vi "QUIZ 1.vi"() -> ()   [LabVIEW 2019]
panel:
  out "Control de pertenencia de la coordenada":bool
  in  "Coordenada Y del punto":dbl[](array[numeric])
  out "Gráfica":T1(graph)
  in  "Coordenada X del punto":dbl[](array[numeric])
  in  "Y polinomio":dbl[](array[numeric])
  in  "X polinomio":dbl[](array[numeric])
  out "By":dbl[](array[numeric])
  out "Bx":dbl[](array[numeric])
  out "Ay":dbl[](array[numeric])
  out "Ax":dbl[](array[numeric])
  out "sum":dbl
  out "Angulos":dbl[](array[numeric])
  # "JOSE IVAN MENDEZ CORREA"
  # "MATEO CARO ROJO"
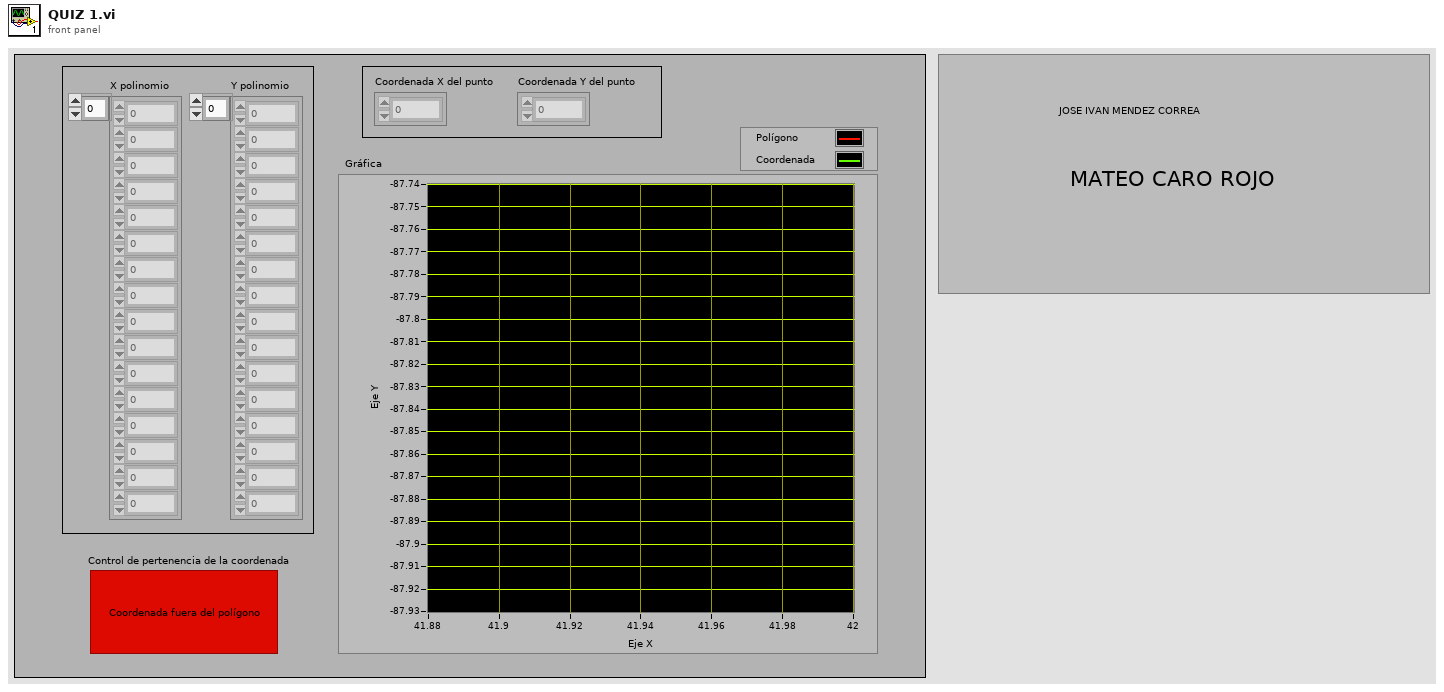
[diagram p1: front panel]
types:
  T1 = cluster{"coordenada X del punto":dbl[], "coordenada y del punto":dbl[]}[]
  T2 = cluster{"X polinomio":dbl[], "Y polinomio":dbl[]}
  T3 = cluster{"Coordenada X del punto":dbl[], "Coordenada Y del punto ":dbl[]}
  T4 = cluster{"Coordenada X del punto":dbl[], "Coordenada Y del punto ":dbl[]}[]
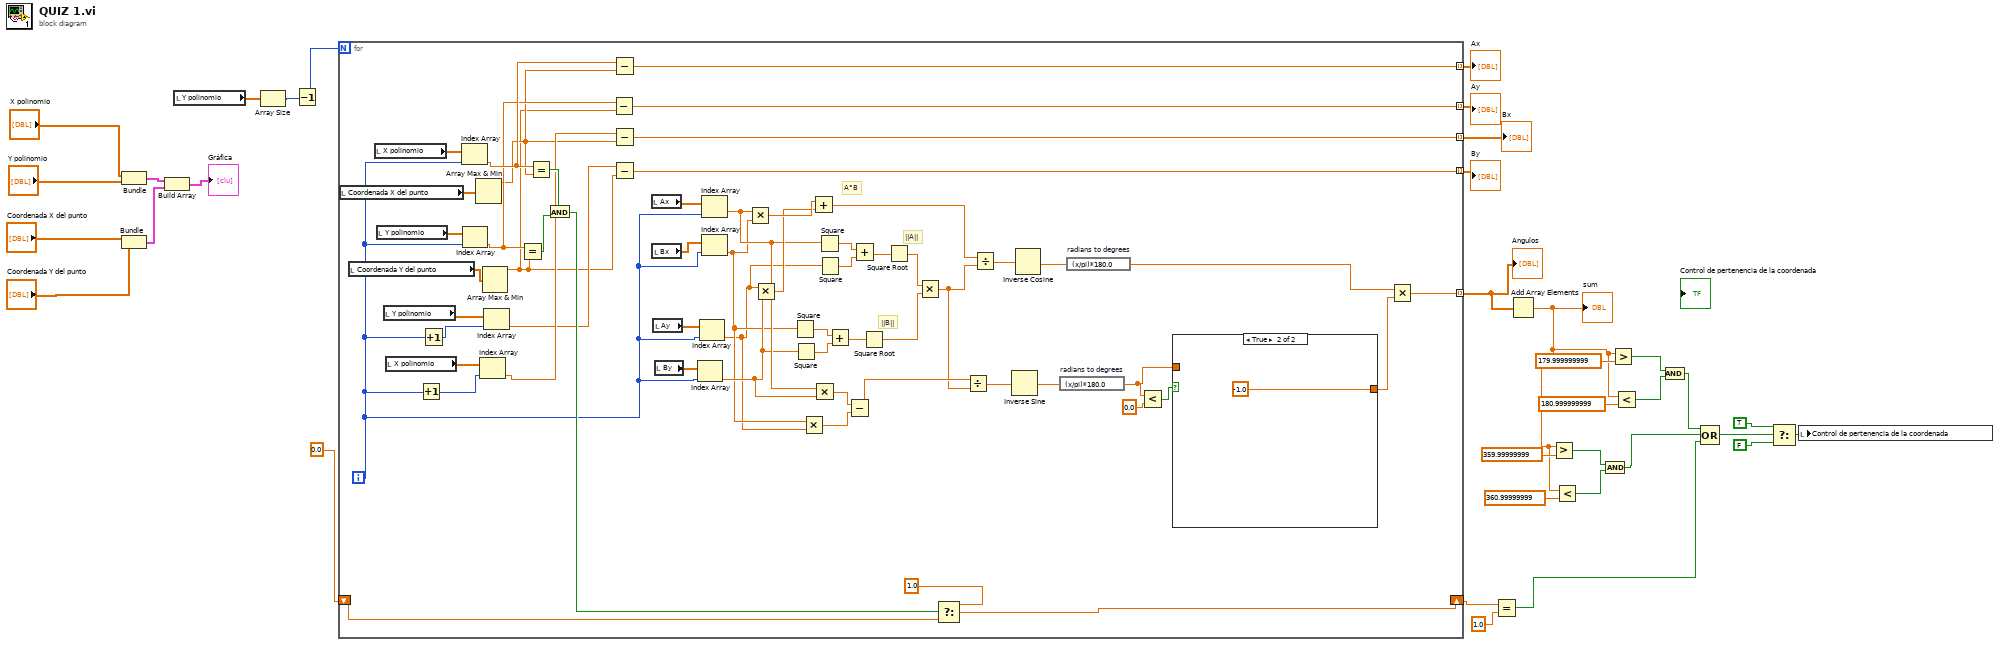
[diagram p0: block diagram]
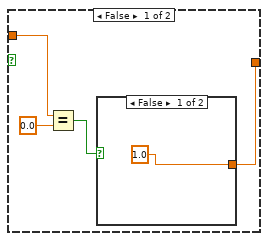
[diagram p2: hidden frame]
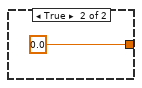
[diagram p3: hidden frame]
diagram:
  n1 = Bundle("X polinomio"="X polinomio", "Y polinomio"="Y polinomio") -> (w32:T2)  [unwired: 1 in]
  n2 = Bundle("Coordenada X del punto"="Coordenada X del punto", "Coordenada Y del punto"="Coordenada Y del punto") -> (w31:T3)  [unwired: 1 in]
  n3 = Build Array(w32, w31) -> (→"Gráfica":T4)
  n4 = local read "Y polinomio"() -> (w27:dbl[])
  n5 = Array Size(array=w27) -> (size(s)=w22:i32)
  n6 = Decrement(x=w22) -> (x-1=w23:i32)
  n7 = for {
    N: w23 -> [_]
    shift-right: [w83] -> w25
    shift-left: 0.0 -> [w86]
    tunnel: [w77] -> w21 mode=indexing
    tunnel: [w75] -> w20 mode=indexing
    tunnel: [w70] -> w19 mode=indexing
    tunnel: [w69] -> w18 mode=indexing
    tunnel: [w35] -> w17 mode=indexing
    i -> [w64]
    # "||B||"
    # "||A||"
    # "A°B"
    n8 = local read "Coordenada X del punto"() -> (w88:dbl[])
    n9 = local read "Coordenada Y del punto"() -> (w87:dbl[])
    n10 = local read "X polinomio"() -> (w92:dbl[])
    n11 = local read "Y polinomio"() -> (w91:dbl[])
    n12 = local read "Y polinomio"() -> (w82:dbl[])
    n13 = local read "X polinomio"() -> (w80:dbl[])
    n14 = Increment(x=w64) -> (x+1=w79:i32)
    n15 = Increment(x=w64) -> (x+1=w81:i32)
    n16 = Index Array(array=w92, index=w64) -> (element=w78:dbl)
    n17 = Index Array(array=w91, index=w64) -> (element=w76:dbl)
    n18 = Array Max & Min(array=w88) -> (max value=w73:dbl)  [unwired: 3 out]
    n19 = Index Array(array=w80, index=w79) -> (element=w74:dbl)
    n20 = Array Max & Min(array=w87) -> (max value=w71:dbl)  [unwired: 3 out]
    n21 = Index Array(array=w82, index=w81) -> (element=w72:dbl)
    n22 = Equal?(x=w76, y=w71) -> (x = y?=w89:bool)
    n23 = Equal?(x=w78, y=w73) -> (x = y?=w90:bool)
    n24 = And(x=w90, y=w89) -> (x .and. y?=w84:bool)
    n25 = Subtract(x=w76, y=w71) -> (x-y=w75:dbl)
    n26 = Subtract(x=w78, y=w73) -> (x-y=w77:dbl)
    n27 = Subtract(x=w74, y=w73) -> (x-y=w70:dbl)
    n28 = Subtract(x=w72, y=w71) -> (x-y=w69:dbl)
    n29 = local read "Ax"() -> (w68:dbl[])
    n30 = local read "Bx"() -> (w67:dbl[])
    n31 = local read "Ay"() -> (w66:dbl[])
    n32 = local read "By"() -> (w65:dbl[])
    n33 = Index Array(array=w65, index=w64) -> (element=w49:dbl)
    n34 = Index Array(array=w66, index=w64) -> (element=w47:dbl)
    n35 = Index Array(array=w68, index=w64) -> (element=w50:dbl)
    n36 = Index Array(array=w67, index=w64) -> (element=w48:dbl)
    n37 = Multiply(x=w50, y=w48) -> (x*y=w63:dbl)
    n38 = Multiply(x=w47, y=w49) -> (x*y=w62:dbl)
    n39 = Square(x=w48) -> (x^2=w58:dbl)
    n40 = Square(x=w49) -> (x^2=w57:dbl)
    n41 = Multiply(x=w48, y=w47) -> (x*y=w45:dbl)
    n42 = Add(x=w63, y=w62) -> (x+y=w53:dbl)
    n43 = Multiply(x=w50, y=w49) -> (x*y=w46:dbl)
    n44 = Square(x=w50) -> (x^2=w61:dbl)
    n45 = Square(x=w47) -> (x^2=w60:dbl)
    n46 = Add(x=w58, y=w57) -> (x+y=w56:dbl)
    n47 = Subtract(x=w46, y=w45) -> (x-y=w44:dbl)
    n48 = Add(x=w61, y=w60) -> (x+y=w59:dbl)
    n49 = Square Root(x=w56) -> (sqrt(x)=w54:dbl)
    n50 = Square Root(x=w59) -> (sqrt(x)=w55:dbl)
    n51 = Multiply(x=w55, y=w54) -> (x*y=w43:dbl)
    n52 = Select(t=1.0, s=w84, f=w86) -> (s? t:f=w83:dbl)
    n53 = Divide(x=w44, y=w43) -> (x/y=w42:dbl)
    n54 = Divide(x=w53, y=w43) -> (x/y=w52:dbl)
    n55 = Inverse Sine(1:w42) -> (0:w41:dbl)
    n56 = Inverse Cosine(1:w52) -> (0:w51:dbl)
    n57 = expression code="(x/pi)*180.0" "radians to degrees"(w41) -> (w38:dbl)
    n58 = expression code="(x/pi)*180.0" "radians to degrees"(w51) -> (w40:dbl)
    n59 = Less?(x=w38, y=0.0) -> (x < y?=w39:bool)
    n60 = case shown="True" w39 {
      tunnel: w38 -> [w96 _]
      tunnel: [w93 -1.0] -> w36
      frame False {
        n61 = Equal?(x=w96, y=0.0) -> (x = y?=w95:bool)
        n62 = case shown="False" w95 {
          tunnel: [1.0 0.0] -> w93
          frame False {
          }
          frame True {
          }
        }
      }
      frame True {
      }
    }
    n63 = Multiply(x=w40, y=w36) -> (x*y=w35:dbl)
  }
  "Angulos" <- w17
  "Ax" <- w21
  "Ay" <- w20
  "Bx" <- w19
  "By" <- w18
  n64 = Equal?(x=w25, y=1.0) -> (x = y?=w1:bool)
  n65 = Add Array Elements(numeric array=w17) -> (sum=w5:dbl)
  "sum" <- w5
  n66 = Greater?(x=w5, y=359.99999999) -> (0:w15:bool)
  n67 = Less?(x=w5, y=360.99999999) -> (x < y?=w13:bool)
  n68 = And(x=w15, y=w13) -> (x .and. y?=w2:bool)
  n69 = Greater?(x=w5, y=179.999999999) -> (0:w8:bool)
  n70 = Less?(x=w5, y=180.999999999) -> (x < y?=w6:bool)
  n71 = And(x=w8, y=w6) -> (x .and. y?=w3:bool)
  n72 = Compound Arithmetic op=OR(w3, w2, w1) -> (w4:bool)
  n73 = Select(t=TRUE, s=w4, f=FALSE) -> (s? t:f=w10:bool)
  n74 = local write "Control de pertenencia de la coordenada"(w10) -> ()
